vi "Test_FGV.vi"() -> ()   [LabVIEW 2017]
uses:
  Command.ctl
panel:
  out "Actual Sample Rate":dbl=1000.0 format="%0.2f"
  in  "stop":bool
  out "Waveform Graph":waveform(dbl)[](graph)
  in  "Daq_ai_para":T1={"Channel"=["Dev01/ai0", "Dev01/ai2"], "Sample rate"=1000.0, "input terminal configuration"=10106} {"input terminal configuration" items=["Default"=-1, "RSE"=10083, "NRSE"=10078, "Differential"=10106, "Pseudodifferential"=12529]}
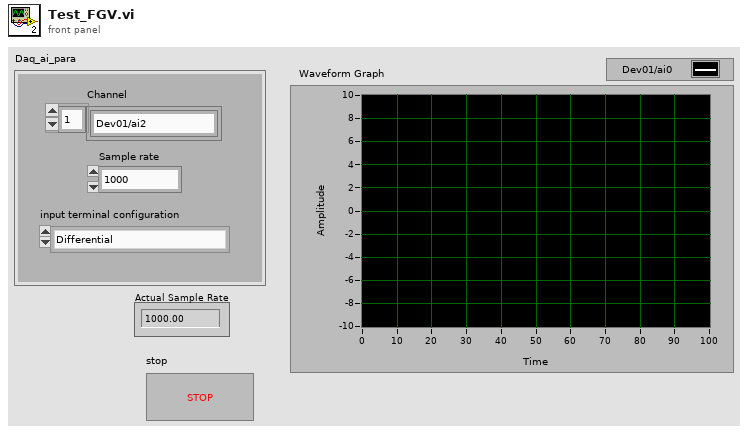
[diagram p1: front panel]
types:
  T1 = cluster{"Channel":string[], "Sample rate":dbl, "input terminal configuration":i32}
  T2 = typedef "Command.ctl" = enum16{"Start Acquire", "Read Data", "Release task"}
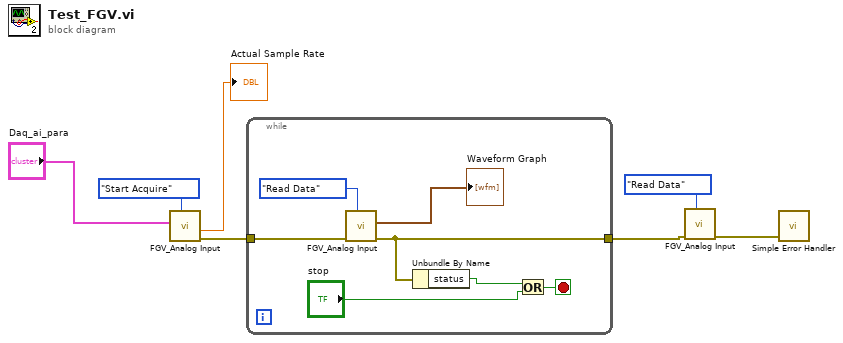
[diagram p0: block diagram]
diagram:
  n1 = call "FGV_Analog Input.vi"("Command"=Command."Start Acquire", "Daq_ai_para"="Daq_ai_para") -> ("error out"=w5:errorcluster, "Actual Sample Rate"=→"Actual Sample Rate":dbl)  [unwired: 7 in, 1 out]
  n2 = while {
    tunnel: w5 -> [w14]
    tunnel: [w11] -> w4
    stop <- w12 stop-if-true
    n3 = call "FGV_Analog Input.vi"("Command"=Command."Read Data", "error in"=w14) -> ("error out"=w11:errorcluster, "data"=→"Waveform Graph":waveform(dbl)[])  [unwired: 7 in, 1 out]
    n4 = Unbundle By Name(w11) -> ("status"=w13:bool)
    n5 = Or(x=w13, y="stop") -> (x .or. y?=w12:bool)
  }
  n6 = call "FGV_Analog Input.vi"("Command"=Command."Read Data", "error in"=w4) -> ("error out"=w2:errorcluster)  [unwired: 7 in, 2 out]
  n7 = call <vilib>:"Simple Error Handler.vi"("error in (no error)"=w2) -> ()  [unwired: 4 in, 5 out]
